vi "To LabVIEW.vi"(4 "TypeMap in":refnum<class "TypeMap.lvclass">, 7 "ExpectedType":refnum<class>, 8 "error in (no error)":errorcluster, 10 "DbRow":variant) -> (0 "error out":errorcluster, 2 "Value":refnum<class>)   [LabVIEW 2020, in "ORM.lvlib" / "TypeMap.lvclass"]
uses:
  TypeMap.lvclass
  TypeMap.lvclass/TypeMap.ctl
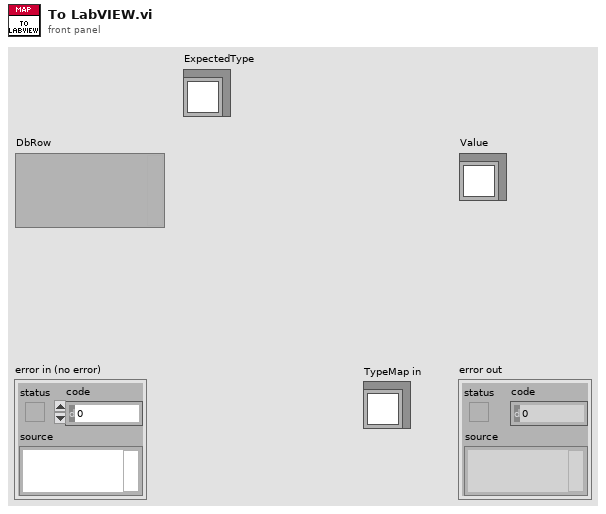
[diagram p1: front panel]
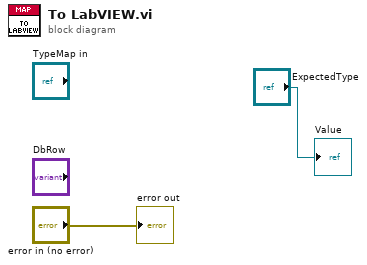
[diagram p0: block diagram]
diagram:
  "error out" <- "error in (no error)"
  "Value" <- "ExpectedType"
